vi "Get_Script_filename.vi"(1 "Traverse line":T1 {"Row Duration (mins)" format="%#.1f"; "Row No" min=0; "Trace Gas Concentration (%)" min=0.0 format="%#.2f"; "Emission Rate (l/min)" format="%#.2f"; "Tunnel Speed" format="%#.2f"; "Start X" format="%#.2f"; "Start Y" format="%#.2f"; "Start Z" format="%#.2f"; "End X" format="%#.2f"; "End Y" format="%#.2f"; "End Z" format="%#.2f"; "Averaging time (min)" min=0.0 format="%#.2f"}) -> (0 "Script Filename":path)   [LabVIEW 2010]
uses:
  Traverse_cluster.ctl
  Spacing.ctl
  Controls/Multi_run_mode.ctl
  Globals/Extra_Commands_Global.vi
  Globals/Constants_global.vi
panel:
  # "X           Y            Z"
  # "Start"
  # "End"
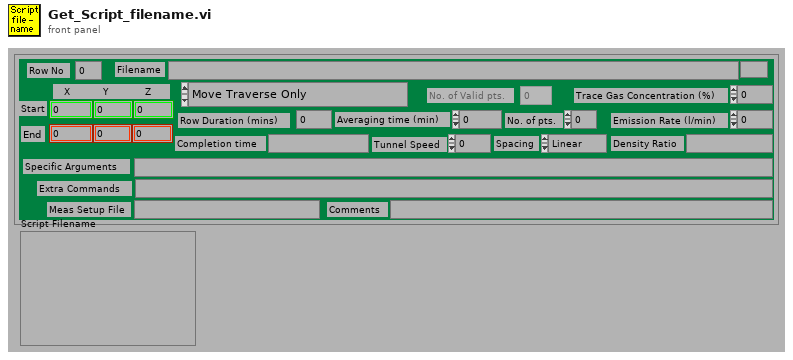
[diagram p1: front panel]
types:
  T1 = typedef "Traverse_cluster.ctl" = cluster{"Start X":dbl, "Start Y":dbl, "Start Z":dbl, "End X":dbl, "End Y":dbl, "End Z":dbl, "No. of pts.":i32, "Spacing":T2, "Filename":path, "Tunnel Speed":dbl, "Averaging time (min)":dbl, "Extra Commands":string, "Specific Arguments":string, "Emission Rate (l/min)":dbl, "Trace Gas Concentration (%)":dbl, "Density Ratio":string, "Comments":string, "Row No":i32, "Row Type Selector":T3, "Completion time":string, "Row Duration (mins)":dbl, "No. of Valid pts.":i32, "Meas Setup File":string}
  T2 = typedef "Spacing.ctl" = enum16{"Linear", "Log", "Gauss", "Specified", "N/A"}
  T3 = typedef "Multi_run_mode.ctl" = enum16{"Move Traverse Only", "Set Tunnel Speed Only", "Set Source Only", "Set Measurement Conditions", "Single Measurement", "Vertical Profile", "Lateral Profile", "Longitudinal Profile", "Explore Volume", "Multi-Axis Profile", "Auto Calibrate", "Meas Fast FID Bkgnd", "Check Beam Power", "Scanning Valve Measurement", "Run VI Named:", "Set ADAM Ch", "Wait (minutes)", "Send Message", "Synchronize With:", "Fall Back to this Row", "Turn Off Row Repeating", "Blank Row"}
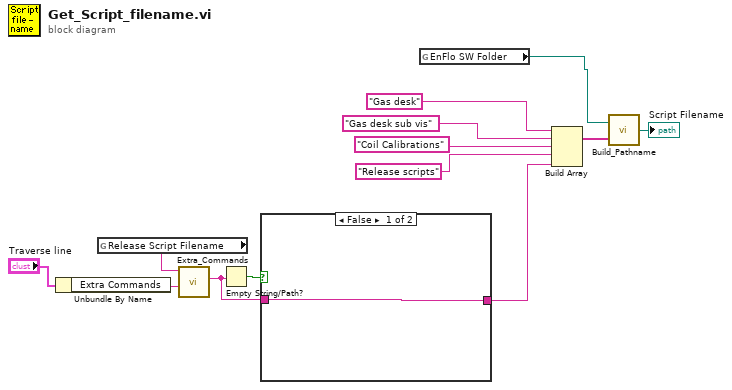
[diagram p0: block diagram]
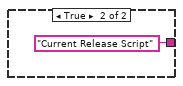
[diagram p2: hidden frame]
diagram:
  n1 = Unbundle By Name("Traverse line") -> ("Extra Commands"=w13:string)
  n2 = global read "Extra_Commands_Global.vi" "Release Script Filename"() -> (w12:string)
  n3 = call "Extra_Commands.vi"("String to Search"=w13, "Command"=w12) -> ("String Value"=w1:string)  [unwired: 1 in, 4 out]
  n4 = Empty String/Path?(string/path=w1) -> (empty?=w2:bool)
  n5 = case shown="False" w2 {
    tunnel: [w14 "Current Release Script"] -> w7
    tunnel: w1 -> [w14 _]
    frame False {
    }
    frame True {
    }
  }
  n6 = global read "Constants_global.vi" "EnFlo SW Folder"() -> (w3:path)
  n7 = Build Array("Gas desk", "Gas desk sub vis", "Coil Calibrations", "Release scripts", w7) -> (w10:string[])
  n8 = call "Build_Pathname.vi"("Output Array"=w10, "Pathname"=w3) -> ("Appended path"=→"Script Filename":path)
